vi "Internet_Checker(MainVI).vi"() -> ()   [LabVIEW 2020]
panel:
  out "error out":errorcluster
  in  "error in":errorcluster
  out "status":bool
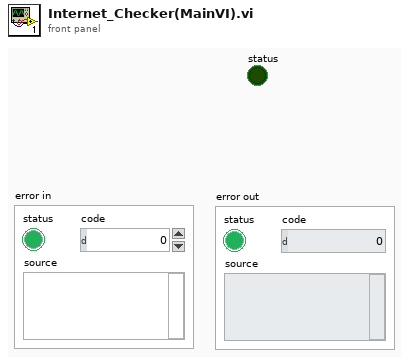
[diagram p1: front panel]
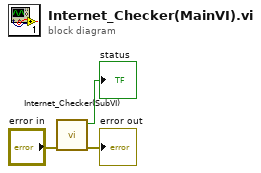
[diagram p0: block diagram]
diagram:
  n1 = call "Internet_Checker(SubVI).vi"("error in (no error)"="error in") -> ("error out"=→"error out":errorcluster, "status"=→"status":bool)  [unwired: 9 in]
